vi "PQfname.vi"(6 "error in (no error)":errorcluster, 7 "cloumn_num":i32, 8 "res":u32) -> (0 "error out":errorcluster, 1 "ColumnName":string, 2 "res_out":u32)   [LabVIEW 2019, in "libpqlv.lvlib"]
doc: "Returns the column name associated with the given column number. Column numbers start at 0. The caller should not free the result directly. It will be freed when the associated PGresult handle is passed to PQclear."
uses:
  libpqlv.lvlib
  libpq.dll
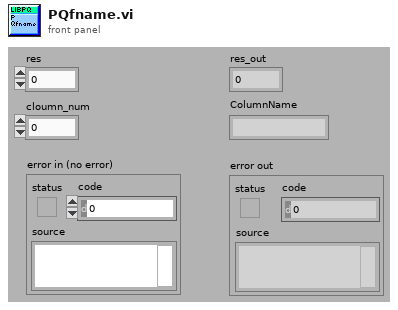
[diagram p1: front panel]
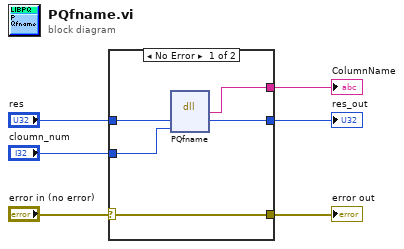
[diagram p0: block diagram]
diagram:
  n1 = case shown="No Error" "error in (no error)" {
    selector: "error in (no error)" -> [w8 w13]
    tunnel: [w8 w13] -> w2
    tunnel: [w11 _] -> w5
    tunnel: "cloumn_num" -> [w10 _]
    tunnel: "res" -> [w9 w12]
    tunnel: [w7 w12] -> w1
    frame No Error {
      n2 = dll-call lib="libpq.*" fn="PQfname"("res"=w9, "field_num"=w10) -> ("col_name"=w11:string, "res"=w7:u32)  [unwired: 4 in, 2 out]
    }
    frame Error {
    }
  }
  "ColumnName" <- w5
  "error out" <- w2
  "res_out" <- w1
